vi "fromXMLNative.vi"(8 "error in (no error)":errorcluster, 10 "scriptEventListXML":refnum<k20>, 11 "ScriptEventList in":refnum<class "ScriptEventList.lvclass">) -> (0 "error out":errorcluster, 3 "ScriptEventList out":refnum<class "ScriptEventList.lvclass">)   [LabVIEW 2011, in "Tools.lvlib" / "Scripting.lvlib" / "ScriptEventList.lvclass"]
uses:
  ScriptEventList.lvclass
  ScriptEventList.lvclass/ScriptEventList.ctl
  <vilib>/xml/Close Reference(Node).vi
  ScriptEvent.lvclass
  <vilib>/xml/NI_XML.lvlib
panel:
  out "open Time":dbl
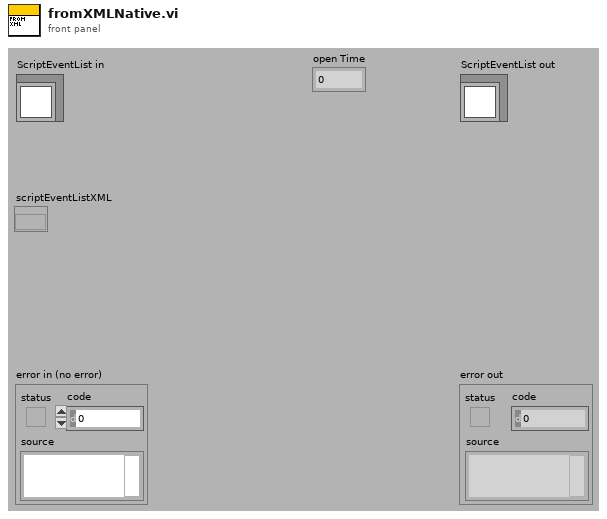
[diagram p1: front panel]
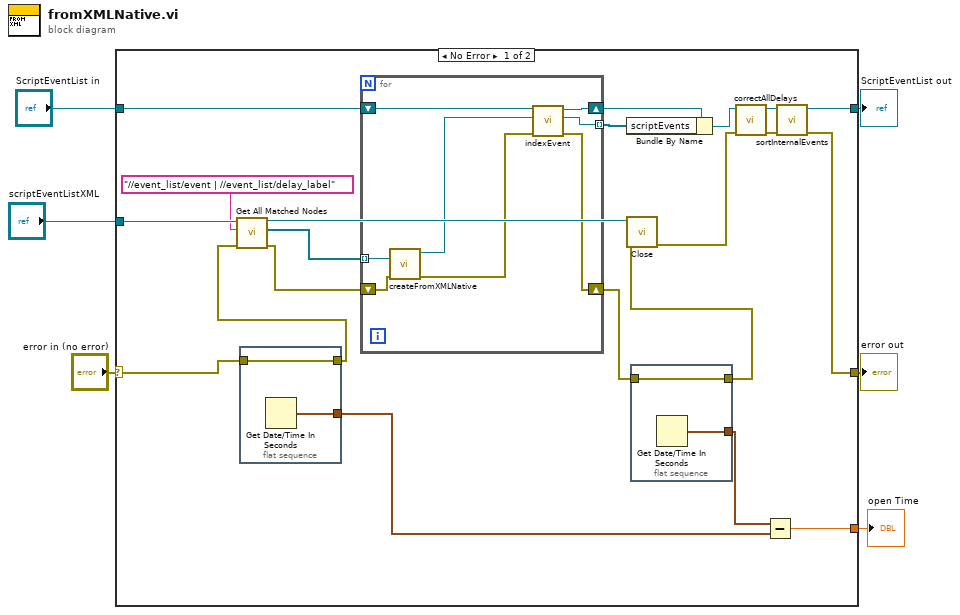
[diagram p0: block diagram]
diagram:
  n1 = case shown="No Error" "error in (no error)" {
    selector: "error in (no error)" -> [w13 w41]
    tunnel: [w15 w41] -> w5
    tunnel: [w16 w40] -> w3
    tunnel: "ScriptEventList in" -> [w22 w40]
    tunnel: "scriptEventListXML" -> [w27 _]
    tunnel: [w7 _] -> w1
    frame No Error {
      n2 = call <vilib>:"Get All Matched Nodes.vi"("error in (no error)"=w12, "XPath expression"="//event_list/event | //event_list/delay_label", "node in"=w27) -> ("error out"=w23:errorcluster, "node result array"=w25:refnum<k20>[], "node out"=w24:refnum<k20>)  [unwired: 6 in]
      n3 = flat-sequence {
        tunnel: [w31] -> w12
        tunnel: w13 -> [w31]
        tunnel: [w30] -> w8
        frame #0 {
          n4 = Get Date/Time In Seconds() -> (seconds since 1Jan1904=w30:timestamp)
        }
      }
      n5 = for {
        tunnel: w25 -> [w36] mode=indexing
        shift-right: [w38] -> w20
        shift-left: w22 -> [w39]
        shift-right: [w37] -> w11
        shift-left: w23 -> [w35]
        tunnel: [w32] -> w21 mode=indexing
        n6 = call "createFromXMLNative.vi"("error in (no error)"=w35, "scriptEventXML"=w36) -> ("error out"=w33:errorcluster, "ScriptEvent out"=w34:refnum<class "ScriptEvent.lvclass">)  [unwired: 8 in]
        n7 = call "indexEvent.vi"("error in (no error)"=w33, "ScriptEvent"=w34, "ScriptEventList in"=w39) -> ("error out"=w37:errorcluster, "ScriptEvent out"=w32:refnum<class "ScriptEvent.lvclass">, "ScriptEventList out"=w38:refnum<class "ScriptEventList.lvclass">)  [unwired: 5 in, 1 out]
      }
      n8 = Bundle By Name(cluster=w20, "scriptEvents"=w21) -> (w17:refnum<class "ScriptEventList.lvclass">)
      n9 = call-poly <vilib>:"Close.vi"("error in (no error)"=w10, "node"=w24) -> ("error out"=w14:errorcluster)  [unwired: 7 in]
      n10 = flat-sequence {
        tunnel: [w29] -> w10
        tunnel: w11 -> [w29]
        tunnel: [w28] -> w9
        frame #0 {
          n11 = Get Date/Time In Seconds() -> (seconds since 1Jan1904=w28:timestamp)
        }
      }
      n12 = call "correctAllDelays.vi"("error in (no error)"=w14, "ScriptEventList in"=w17) -> ("error out"=w18:errorcluster, "ScriptEventList out"=w19:refnum<class "ScriptEventList.lvclass">)  [unwired: 8 in]
      n13 = Subtract(x=w9, y=w8) -> (x-y=w7:dbl)
      n14 = call "sortInternalEvents.vi"("error in (no error)"=w18, "ScriptEventList in"=w19) -> ("error out"=w15:errorcluster, "ScriptEventList out"=w16:refnum<class "ScriptEventList.lvclass">)  [unwired: 8 in]
    }
    frame Error {
    }
  }
  "error out" <- w5
  "ScriptEventList out" <- w3
  "open Time" <- w1
